vi "test_HostApi Error because big Sec wait time .vi"(8 "error in (no error)":errorcluster) -> (0 "error out":errorcluster)   [LabVIEW 2019, in "Host API Tests.lvclass"]
uses:
  Host API Tests.lvclass
  Addon/Addon Shared/Types/Buffered RT Instrument Command.ctl
  Addon/Addon Shared/Types/Response Wait Type.ctl
  <vilib>/addons/_JKI Toolkits/VI Tester/TestCase.llb/TestCase.lvclass
  APIs/Host Automation API/Instrument Host Automation API.lvlib
  Addon/Addon Shared/Instrument Addon Shared.lvlib
  C:/Program Files (x86)/National Instruments/LabVIEW 2019/vi.lib/addons/_JKI Toolkits/VI Tester/TestCase.llb/TestCase.lvclass
panel:
  out "TestCase out":refnum<class "Host API Tests.lvclass">
  in  "TestCase in":refnum<class "Host API Tests.lvclass">
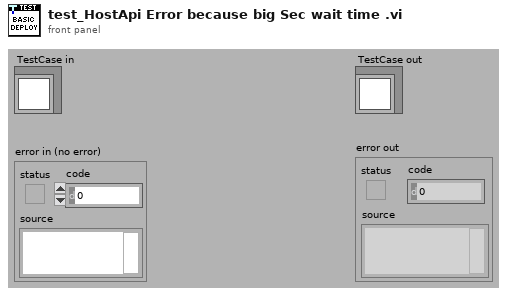
[diagram p1: front panel]
types:
  T1 = typedef "Instrument Addon Shared.lvlib/Buffered RT Instrument Command.ctl" = cluster{"Command":string, "Response Expected?":bool, "Wait Type":T2, "Wait Value":dbl}
  T2 = typedef "Instrument Addon Shared.lvlib/Response Wait Type.ctl" = enum16{"Byte Count", "Wait sec"}
  T3 = typedef "NI STM.lvlib/TCP Connection Info.ctl" = cluster{"connection ID":refnum<k5>, "meta data":T4[]}
  T4 = typedef "NI STM.lvlib/MetaDataElement.ctl" = string
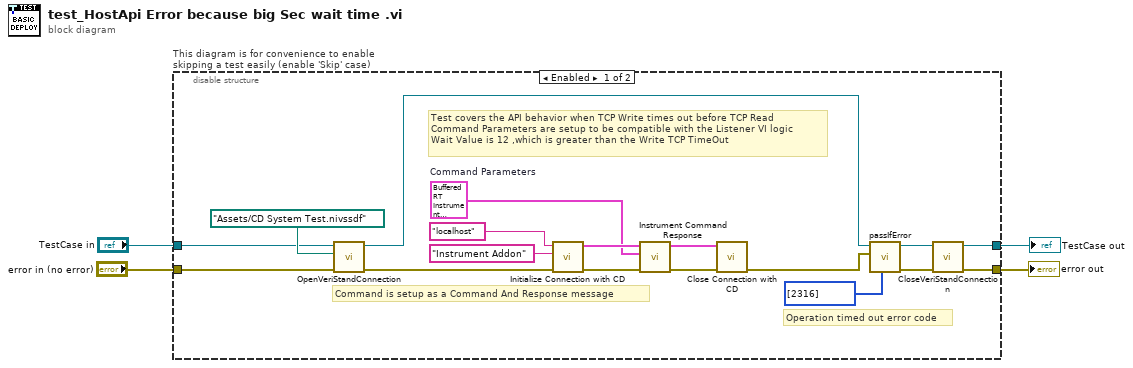
[diagram p0: block diagram]
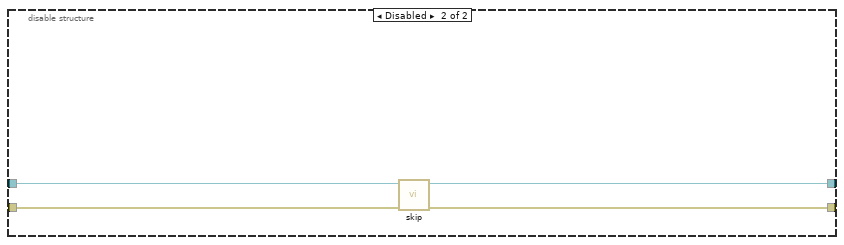
[diagram p2: hidden frame]
diagram:
  n1 = disable-structure "This diagram is for convenience to enable skipping a test easily (enable 'Skip' case)" shown="Enabled" {
    disable-tunnel: "TestCase in" -> [w20 w26]
    disable-tunnel: [w18 w24] -> w1
    disable-tunnel: [w19 w25] -> w3
    disable-tunnel: "error in (no error)" -> [w21 w23]
    frame Enabled {
      w7 = T1 {"Command"="22LabVIEWCommandResponse", "Response Expected?"=TRUE, "Wait Type"=enum."Wait sec", "Wait Value"=12.0}  # Command Parameters
      # "Operation timed out error code"
      # "Test covers the API behavior when TCP Write times out before TCP Read\nCommand Parameters are setup to be compatible with the Listener VI logic\nWait Value is 12 ,which is greater than the Write TCP TimeOut"
      # "Command is setup as a Command And Response message"
      n2 = call-dynamic "OpenVeriStandConnection.vi"("error in (no error)"=w21, "System Definition File"=path "Assets/CD System Test.nivssdf", "VeriStand Test Case in"=w20) -> ("error out"=w8:errorcluster, "VeriStand Test Case out"=w16:refnum<class "Host API Tests.lvclass">)  [unwired: 6 in, 1 out]
      n3 = call "Initialize Connection with CD.vi"("error in (no error)"=w8, "TCP Service"="Instrument Addon", "IP Address"="localhost") -> ("error out"=w12:errorcluster, "connection info out"=w11:T3)  [unwired: 7 in]
      n4 = call "Instrument Command Response.vi"("error in (no error)"=w12, "Command Parameters"=w7, "Comm.Info"=w11) -> ("error out"=w10:errorcluster, "Comm.Info"=w9:T3)  [unwired: 5 in, 2 out]
      n5 = call "Close Connection with CD.vi"("error in"=w10, "Comm.Info"=w9) -> ("error out"=w5:errorcluster)  [unwired: 9 in]
      n6 = call-dynamic "passIfError.vi"("passing error codes (default = any error code)"=i32[] [2316], "error"=w5, "TestCase in"=w16) -> ("error out"=w17:errorcluster, "TestCase out"=w15:refnum<class "Host API Tests.lvclass">)  [unwired: 7 in]
      n7 = call-dynamic "CloseVeriStandConnection.vi"("error in (no error)"=w17, "VeriStand Test Case in"=w15) -> ("error out"=w19:errorcluster, "VeriStand Test Case out"=w18:refnum<class "Host API Tests.lvclass">)  [unwired: 8 in]
    }
    frame Disabled {
      # "skip test result while test is under development"
      n8 = call <vilib>:"skip.vi"("error in (no error)"=w23, "TestCase in"=w26) -> ("error out"=w25:errorcluster, "TestCase out"=w24:refnum<class "Host API Tests.lvclass">)  [unwired: 8 in]
    }
  }
  "error out" <- w3
  "TestCase out" <- w1
